vi "Main_FGV_Data.vi"(7 "Action_Data":T1, 10 "Data In":cluster{"Data name":string, "Data":variant}, 11 "Data name":string) -> (1 "Data Array out":cluster{"Data name":string, "Data":variant}[](array[cluster]), 2 "Data  Out":cluster{"Data name":string, "Data":variant})   [LabVIEW 2015]
uses:
  Control/Action_Data.ctl
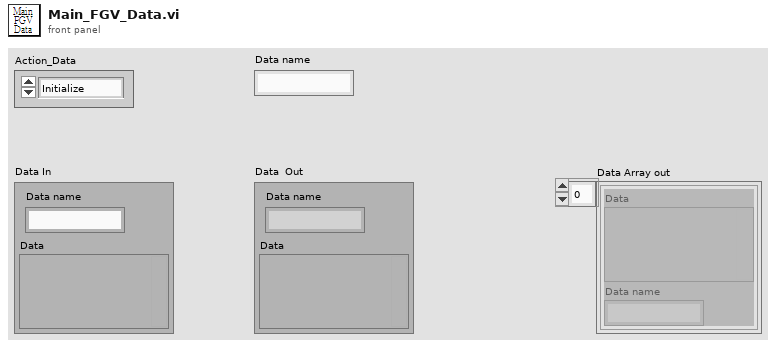
[diagram p1: front panel]
types:
  T1 = typedef "Action_Data.ctl" = enum16{"Initialize", "Get Data", "Set Data", "Delete Data", "Idle"}
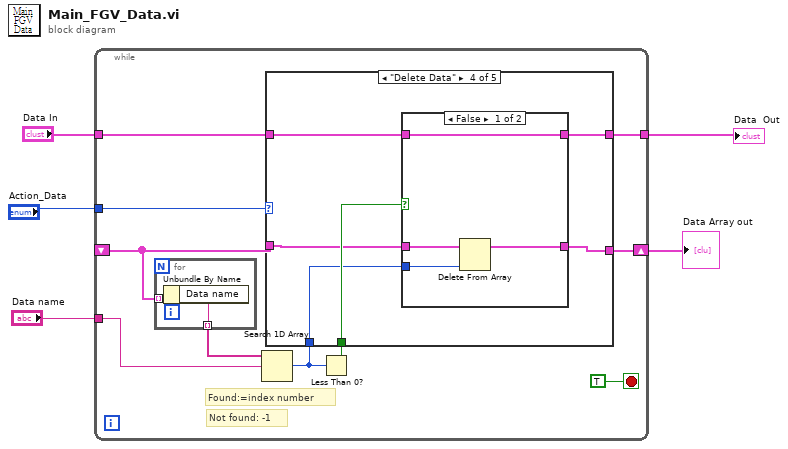
[diagram p0: block diagram]
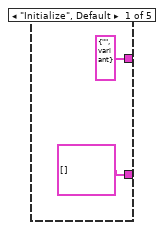
[diagram p2: hidden frame]
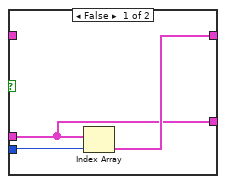
[diagram p4: hidden frame]
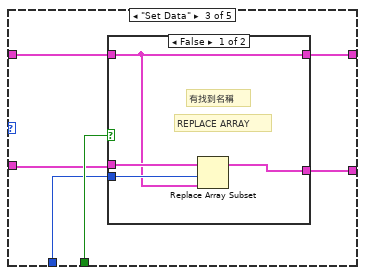
[diagram p5: hidden frame]
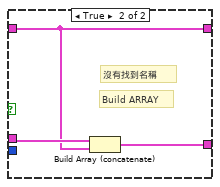
[diagram p6: hidden frame]
diagram:
  n1 = while {
    tunnel: "Action_Data" -> [w15]
    tunnel: "Data In" -> [w13]
    tunnel: [w12] -> w2
    shift-right: [w11] -> w1
    shift-left: _ -> [w10]
    tunnel: "Data name" -> [w8]
    stop <- TRUE stop-if-true
    # "Not found: -1"
    # "Found:=index number"
    n2 = for {
      tunnel: w10 -> [w17] mode=indexing
      tunnel: [w16] -> w9 mode=indexing
      n3 = Unbundle By Name(w17) -> ("Data name"=w16:string)
    }
    n4 = Search 1D Array(1D array=w9, element=w8) -> (index of element=w6:i32)  [unwired: 1 in]
    n5 = Less Than 0?(x=w6) -> (x < 0?=w7:bool)
    n6 = case shown="\"Delete Data\"" w15 {
      tunnel: w13 -> [_ w20 w31 w44 w57]
      tunnel: [cluster{"Data name":string, "Data":variant} {"Data name"="", "Data"=variant} ("Data In") w22 w32 w45 w57] -> w12
      tunnel: [cluster{"Data name":string, "Data":variant}[] [] w21 w33 w46 w56] -> w11
      tunnel: w10 -> [_ w24 w34 w48 w56]
      tunnel: w7 -> [_ w25 w36 w49 _]
      tunnel: w6 -> [_ w23 w35 w47 _]
      frame "Initialize", Default {
      }
      frame "Get Data" {
        n7 = case shown="True" w25 {
          tunnel: w24 -> [w26 w30]
          tunnel: w23 -> [w28 _]
          tunnel: [w27 w29] -> w22
          tunnel: [w26 w30] -> w21
          tunnel: w20 -> [_ w29]
          frame False {
            n8 = Index Array(array=w26, index=w28) -> (element=w27:cluster{"Data name":string, "Data":variant})
          }
          frame True {
          }
        }
      }
      frame "Set Data" {
        n9 = case shown="False" w36 {
          tunnel: w35 -> [w40 _]
          tunnel: w34 -> [w39 w43]
          tunnel: [w38 w42] -> w33
          tunnel: [w37 w41] -> w32
          tunnel: w31 -> [w37 w41]
          frame False {
            # "REPLACE ARRAY"
            # "有找到名稱"
            n10 = Replace Array Subset(array=w39, new element=w37, index=w40) -> (w38:cluster{"Data name":string, "Data":variant}[])
          }
          frame True {
            # "Build ARRAY"
            # "沒有找到名稱"
            n11 = Build Array (concatenate)(w43, w41) -> (w42:cluster{"Data name":string, "Data":variant}[])
          }
        }
      }
      frame "Delete Data" {
        n12 = case shown="False" w49 {
          tunnel: w48 -> [w53 w55]
          tunnel: w47 -> [w50 _]
          tunnel: [w52 w55] -> w46
          tunnel: [w51 w54] -> w45
          tunnel: w44 -> [w51 w54]
          frame False {
            n13 = Delete From Array(array=w53, index=w50) -> (array with subset deleted=w52:cluster{"Data name":string, "Data":variant}[])  [unwired: 1 in, 1 out]
          }
          frame True {
          }
        }
      }
      frame "Idle" {
      }
    }
  }
  "Data  Out" <- w2
  "Data Array out" <- w1
